vi "Find Valid in String.vi"(11 "string":string) -> (2 "number of findings":i32, 3 "Found":bool)   [LabVIEW 2024]
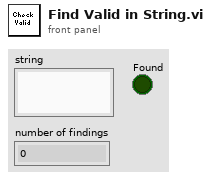
[diagram p1: front panel]
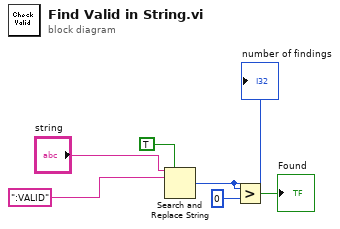
[diagram p0: block diagram]
diagram:
  n1 = Search and Replace String(replace all?=TRUE ("replace all? (F)"), input string="string", search string=":VALID") -> (number of replacements=w4:i32)  [unwired: 5 in, 3 out]
  "number of findings" <- w4
  n2 = Greater?(x=w4, y=0) -> (0:→"Found":bool)
